vi "4_Speech_Rec_Deploy(mic).vi"() -> ()   [LabVIEW 2020]
doc: "This example demonstrates the usage of Deep Learning Toolkit for loading the model pretrained for objects recognition and running for inference."
uses:
  <vilib>/Ngene/Deep Learning Toolkit/Toolkit/NN_Network/Controls/NN_Device.ctl
  <vilib>/Ngene/Deep Learning Toolkit/Toolkit/NN_Network/Controls/NN_Save_Before_Destroy_Options.ctl
  <vilib>/sound2/lvsound2.llb/Sampling Mode.ctl
  <vilib>/sound2/lvsound2.llb/Sound Data Format.ctl
  <vilib>/Analysis/5stat.llb/RMS (DBL).vi
  <vilib>/sound2/lvsound2.llb/Sound Input Read (DBL).vi
  <vilib>/Ngene/Deep Learning Toolkit/Toolkit/NN_Network/API/NN_Set_Input/3D/NN_Set_Input(3D_SGL_idx).vi
  <vilib>/Ngene/Deep Learning Toolkit/Toolkit/Deep_Learning_Toolkit_by_Ngene.lvlib
  <vilib>/vision/NI_Vision_Development_Module.lvlib
  <vilib>/Analysis/NI_AALPro.lvlib
panel:
  out "Spectrogram":dbl[][](graph)
  out "Class Labels":string[](array[string])=["no", "stop", "down", "dog", "backward", "sheila", "zero", "visual", "wow", "left", "nine", "learn", "one", "go", "yes", "up", "follow", "four", "cat", "seven", "two", "_background_noise_", "off", "happy", "right", "bed", "marvin", "five", "six", "forward", "bird", "tree", "eight", "three", "house", "on"]
  out "Waveform":waveform(dbl)(graph)={"t0"=timestamp(3866543015.0437703 s since 1904-01-01), "dt"=6.25e-05, "Y"=array[16000 elements]}
  out "Class Probabilities":sgl[](array[slide])=[0.3439477, 0.21329805, 0.094255894, 0.046067823, 0.04473784, 0.04242303, 0.03942926, 0.036859456, 0.03191309, 0.028905181, 0.027009873, 0.013410927, 0.011738547, 0.0056317565, 0.005620018, 0.00169456, 0.00161148, 0.0014156047, 0.0013186012, 0.0013032081, 0.0012892308, 0.0008470631, 0.0008419843, 0.00080975075, 0.0006212335, 0.00061424717, 0.00059279194, 0.000582364, 0.00025428596, 0.00022874227, 0.0001889991, 0.00015415151, 0.00014091097, 0.00012097955, 6.820219e-05, 5.3142972e-05] scale=0.0..1.0
  in  "NN Device":T1=enum."GPU"
  out "Inference Time(sec)":dbl=0.012933300007716753 format="%#_3p"
  in  "Network Configuration File Path":path=path "D:/working/speech_rec/Speech_Rec_net_cfg_26_07_10__17_58_19.cfg"
  in  "Weight File Path":path=path "D:/working/speech_rec/Speech_Rec_weights_26_07_10__17_58_19.bin"
  in  "Stop":bool
  in  "threshold":dbl=0.01 format="%#_13g"
  # "Overview: This example demonstrates the use of Deep Learning Toolkit for loading a model pretrained for speech recognition and running it for inference.\nRequirements:\n1. Deep Learning Toolkit for LabVIEW.\n2. NI Vision Development Module.\n3. A PC with audio input (microphone).\nInstructions:\nThis example requires the trained model (network topology file .cfg and trained weights file .bin) generated in the previous step.\n1. Provide the trained model files at \"Network Configuration File Path\" and \"Weight File Path\".\n2. Run the VI.\n3. Pronounce one of the words from the dataset and observe the prediction results.\n4. Adjust the threshold value to reduce the false detection rate or increase sensitivity."
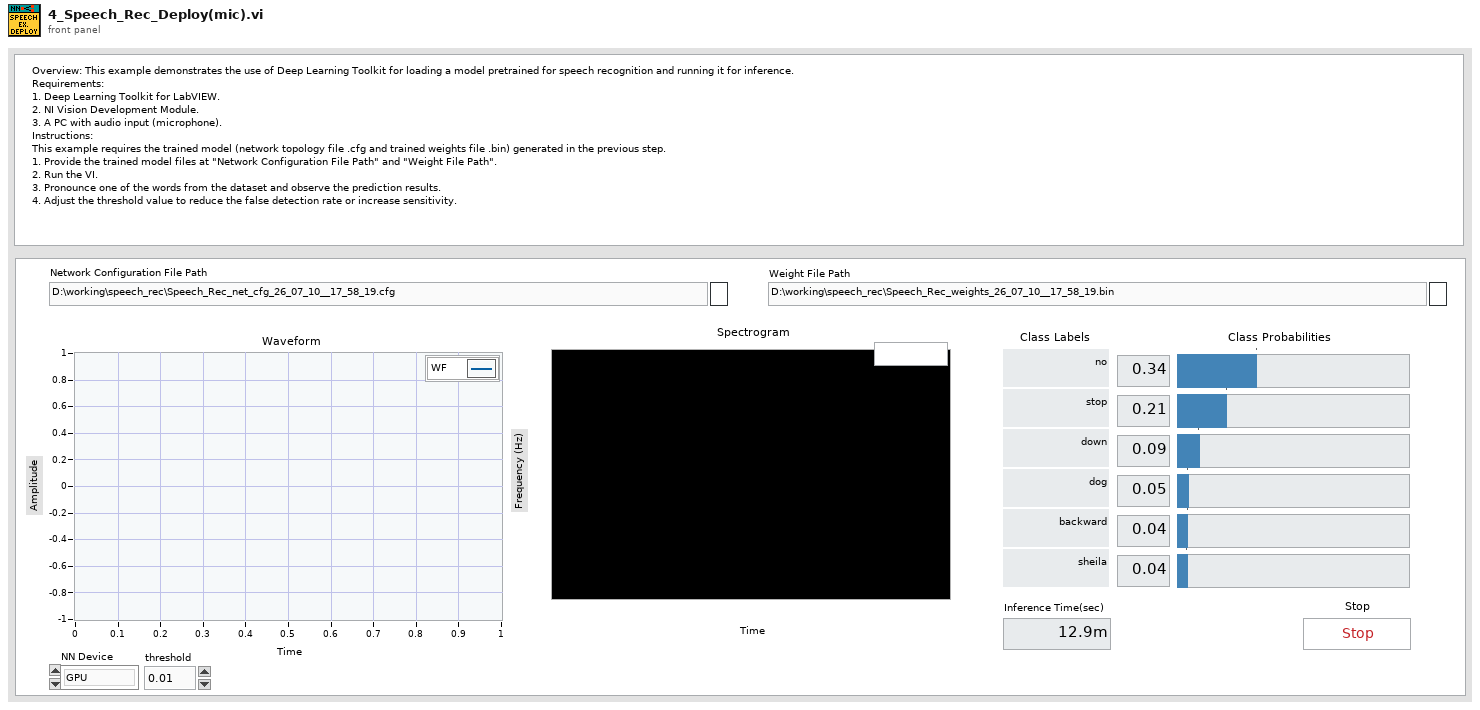
[diagram p1: front panel]
types:
  T1 = typedef "Deep_Learning_Toolkit_by_Ngene.lvlib/NN_Device.ctl" = enum16{"CPU", "GPU"}
  T2 = typedef "Sound Data Format.ctl" = cluster{"sample rate (S/s)":dbl, "number of channels":i32, "bits per sample":i32}
  T3 = typedef "Sampling Mode.ctl" = i32
  T4 = typedef "Image Type" = u32
  T5 = typedef "Deep_Learning_Toolkit_by_Ngene.lvlib/NN_Save_Before_Destroy_Options.ctl" = cluster{"CFG?":bool, "Weights?":bool, "Render?":bool}
  T6 = typedef "Sound Input Task ID.ctl" = u32
  T7 = typedef "Deep_Learning_Toolkit_by_Ngene.lvlib/NN_Config_Params.ctl" = cluster{"Name":string, "mBatch":i32, "NN_Train_Params":T8, "LR_Decay_Policy":T11, "Labels":string[], "Loss":T13, "Max_WS_Size(B)":i64, "DryRun?":bool}
  T8 = typedef "Deep_Learning_Toolkit_by_Ngene.lvlib/NN_Train_Params.ctl" = cluster{"Optimizer":T9, "Beta_1":sgl, "Beta_2":sgl, "Weight Decay(L1)":sgl, "Weight Decay(L2)":sgl, "Data_Sampling":T10}
  T9 = typedef "Deep_Learning_Toolkit_by_Ngene.lvlib/NN_Train_Optimizer.ctl" = enum16{"SGD", "Adam", "Adagrad", "Adadelta", "RMSProp", "Nesterov"}
  T10 = typedef "Deep_Learning_Toolkit_by_Ngene.lvlib/NN_Train_Data_Sampling.ctl" = enum16{"Random", "Sequential"}
  T11 = typedef "Deep_Learning_Toolkit_by_Ngene.lvlib/NN_LR_Policy_Cfg.ctl" = cluster{"Policy_Type":T12, "LR0":dbl, "k":sgl, "WarmUp_Policy":enum16{"Step", "Ramp"}, "WarmUp_Iter":i32, "WarmUp_Ratio":sgl}
  T12 = typedef "Deep_Learning_Toolkit_by_Ngene.lvlib/NN_LR_Policy_Type.ctl" = enum16{"Manual", "Step", "Exp", "1/t"}
  T13 = typedef "Deep_Learning_Toolkit_by_Ngene.lvlib/NN_Loss_Config_Params.ctl" = cluster{"Loss_Type":T14, "Loss_Conf_Params":variant}
  T14 = typedef "Deep_Learning_Toolkit_by_Ngene.lvlib/NN_Loss_Type.ctl" = enum16{"None", "MSE", "CrossEntropy", "YOLO_v2", "YOLO_v4"}
  T15 = typedef "Deep_Learning_Toolkit_by_Ngene.lvlib/NN_Layer_Config_Params.ctl" = cluster{"Layer_Type":T16, "Layer_Conf_Params":variant, "Input Layers":string[]}
  T16 = typedef "Deep_Learning_Toolkit_by_Ngene.lvlib/NN_Layer_Type.ctl" = enum16{"Input1D", "Input3D", "Conv1D", "Conv2D", "Conv2D_Adv", "MaxPool", "AvgPool", "UpSample", "DropOut3D", "ShortCut", "Concat", "SoftMax3D", "FC", "DropOut", "Softmax", "Flatten", "YOLO_v2", "YOLO_v4", "Activation", "BatchNormalization", "LayerNormalization", "Scale", "Unsupported"}
  T17 = typedef "Deep_Learning_Toolkit_by_Ngene.lvlib/NN.ctl" = cluster{"Name":string, "No of Layers":i32, "mBatch":i32, "Layers":T18[], "Dimty":T19, "Dims_In":T20, "Dims_Out":T20, "Working_Dir":path, "Train?":bool, "Train_Params":T8, "LR_Update_Policy":T11, "Session Data":T21, "Ground_truth":T22, "NNg_hdls":T23, "NN_Device":T1, "GPU Id":i32, "Labels":string[], "Loss_Type":T14, "Loss_Cfg_Prms":variant, "NNG_WS":T24, "DryRun?":bool}
  T18 = typedef "Deep_Learning_Toolkit_by_Ngene.lvlib/NN_Layer_ref.ctl" = refnum<file>
  T19 = typedef "Deep_Learning_Toolkit_by_Ngene.lvlib/NN_In_Out_Dim-ty.ctl" = enum8{"In1D_Out1D", "In3D_Out1D", "In3D_Out3D", "In3D_OutBBox"}
  T20 = typedef "Deep_Learning_Toolkit_by_Ngene.lvlib/NN_Dims(C,H,W).ctl" = cluster{"C":i32, "H":i32, "W":i32}
  T21 = typedef "Deep_Learning_Toolkit_by_Ngene.lvlib/NN_Train_Session_Data.ctl" = cluster{"Epochs":sgl, "Tot_Iter":i32, "LR":sgl, "LR_iter":i32}
  T22 = typedef "Deep_Learning_Toolkit_by_Ngene.lvlib/NN_Ground_truth.ctl" = cluster{"Y":variant}
  T23 = typedef "Deep_Learning_Toolkit_by_Ngene.lvlib/nng_cuda_handles.ctl" = cluster{"cudnn":u64, "cublas":u64, "stream":u64, "curand":u64}
  T24 = typedef "Deep_Learning_Toolkit_by_Ngene.lvlib/NNG_WS.ctl" = cluster{"NNG_WS_Mem":T25, "Max_WS_Size":i64}
  T25 = typedef "Deep_Learning_Toolkit_by_Ngene.lvlib/NNg_WS_Mem_DVR.ctl" = refnum<data-value>
  T26 = typedef "IMAQ Image.ctl" = refnum<image>
  T27 = cluster{"spectral map":dbl[][], "X scale":cluster{"offset":dbl, "multiplier":dbl}, "Y scale":cluster{"offset":dbl, "multiplier":dbl}, "attribute":variant}
  T28 = typedef "Deep_Learning_Toolkit_by_Ngene.lvlib/NN_Layer.ctl" = cluster{"Name":string, "Layer_Data":T29, "Layer_Type":T16, "Dims_In":T20, "Layers_In":T18[], "Dims_Out":T20, "Layers_Out":T18[], "Metrics":T30, "GPU_Data":T31, "mBatch":i32, "NN_Device":T1, "NNg_hdls":T23, "Train?":bool, "Dimty":T32, "RecptField":T33, "Idx":i32}
  T29 = typedef "Deep_Learning_Toolkit_by_Ngene.lvlib/NN_Layer_Data_Refnum.ctl" = refnum<file>
  T30 = typedef "Deep_Learning_Toolkit_by_Ngene.lvlib/NN_Layer_Metrics.ctl" = cluster{"Data":dbl, "Params":dbl, "Ops":dbl}
  T31 = typedef "Deep_Learning_Toolkit_by_Ngene.lvlib/NNg_Layer_Data_Refnum.ctl" = refnum<file>
  T32 = typedef "Deep_Learning_Toolkit_by_Ngene.lvlib/NN_Layer_Dimty.ctl" = enum16{"1D", "3D"}
  T33 = typedef "Deep_Learning_Toolkit_by_Ngene.lvlib/NN_Layer_RF_State.ctl" = cluster{"Dims":T34, "J":T34}
  T34 = typedef "Deep_Learning_Toolkit_by_Ngene.lvlib/NN_Dims(V,H).ctl" = cluster{"V":i32, "H":i32}
  T35 = cluster{"Numeric Control":sgl, "Labels":string}[]
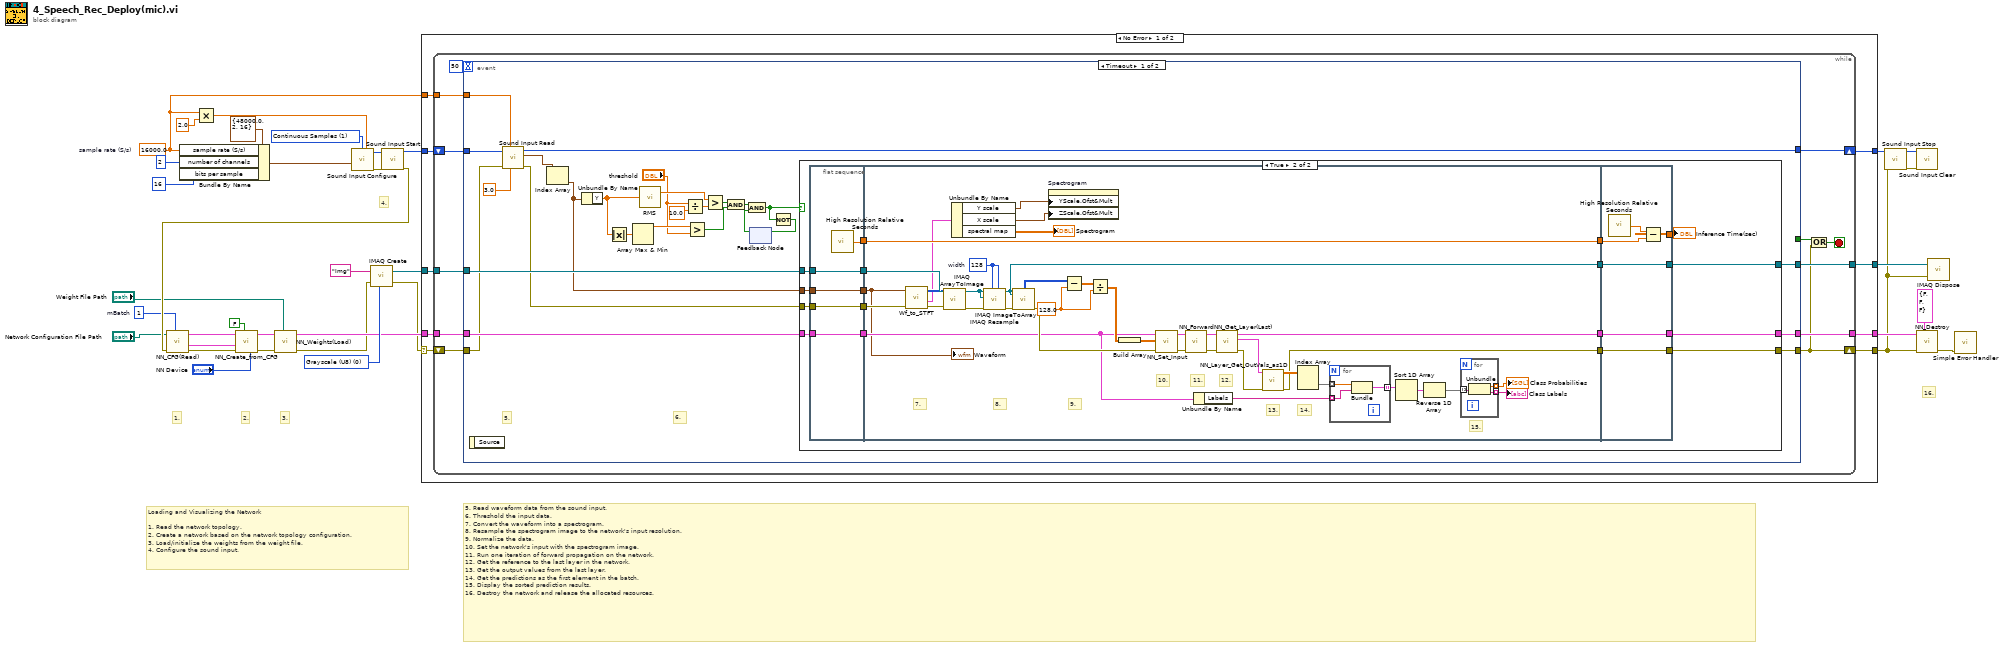
[diagram p0: block diagram]
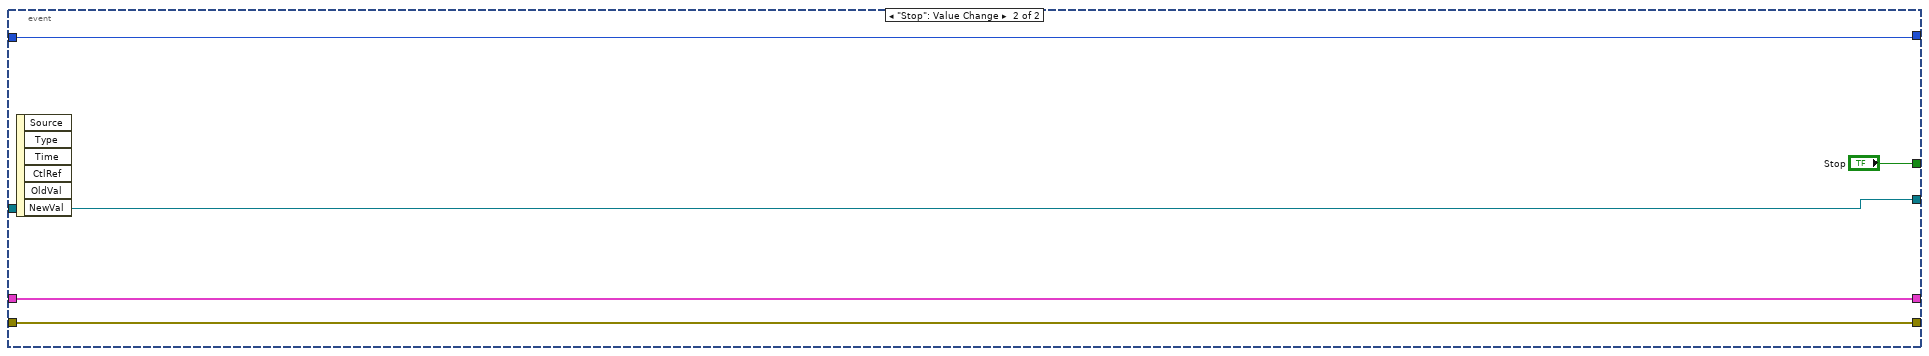
[diagram p3: hidden frame]
diagram:
  w4 = 1  # mBatch
  w9 = 16000.0  # sample rate (S/s)
  w18 = T3 1 items=["Finite Samples", "Continuous Samples"] ("sample mode")
  w32 = T4 0 items=["Grayscale (U8)", "Grayscale (I16)", "Grayscale (SGL)", "Complex (CSG)", "RGB (U32)", "HSL (U32)", "RGB (U64)", "Grayscale (U16)"] ("Image Type")
  # "16."
  # "5. Read waveform data from the sound input.\n6. Threshold the input data.\n7. Convert the waveform into a spectrogram.\n8. Resample the spectrogram image to the network's input resolution.\n9. Normalize the data.\n10. Set the network's input with the spectrogram image.\n11. Run one iteration of forward propagation on the network.\n12. Get the reference to the last layer in the network.\n13. Get the output values from the last layer.\n14. Get the predictions as the first element in the batch.\n15. Display the sorted prediction results.\n16. Destroy the network and release the allocated resources."
  # "4."
  # "3."
  # "2."
  # "1."
  # "Loading and Visualizing the Network\n\n1. Read the network topology.\n2. Create a network based on the network topology configuration.\n3. Load/initialize the weights from the weight file.\n4. Configure the sound input."
  n1 = Bundle By Name(cluster=T2 {"sample rate (S/s)"=48000.0, "number of channels"=2, "bits per sample"=16} ("sound format"), "sample rate (S/s)"=w9, "number of channels"=2, "bits per sample"=16) -> (w20:T2)
  n2 = Multiply(x=w9, y=2.0 ("x")) -> (x*y=w10:dbl)
  n3 = call <vilib>:"Sound Input Configure.vi"("number of samples/ch"=w10, "sample mode"=w18, "sound format"=w20) -> ("error out"=w17:errorcluster, "task ID"=w16:T6)  [unwired: 7 in]
  n4 = call <vilib>:"Sound Input Start.vi"("error in (no error)"=w17, "task ID"=w16) -> ("error out"=w6:errorcluster, "task ID out"=w15:T6)  [unwired: 8 in]
  n5 = call <vilib>:"NN_CFG(Read).vi"("mBatch"=w4, "error in (no error)"=w6, "CFG file path"="Network Configuration File Path") -> ("error out"=w30:errorcluster, "Net_Cfg"=w29:T7, "Layer_Cfg"=w8:T15[])  [unwired: 6 in]
  n6 = call <vilib>:"NN_Create_from_CFG.vi"("NN_Device"="NN Device", "Train? (false)"=FALSE, "error in (no error)"=w30, "Net_Cfg"=w29, "Layer_Cfg"=w8) -> ("error out"=w28:errorcluster, "NN out"=w7:T17)  [unwired: 5 in]
  n7 = call <vilib>:"NN_Weights(Load).vi"("Weight File Path"="Weight File Path", "error in (no error)"=w28, "NN in"=w7) -> ("error out"=w24:errorcluster, "NN out"=w27:T17)  [unwired: 7 in]
  n8 = call "IMAQ Create"("Image Name"="Img", "Image Type"=w32, "error in (no error)"=w24) -> ("New Image"=w31:T26, "error out"=w23:errorcluster)  [unwired: 2 in]
  n9 = case shown="No Error" w23 {
    selector: w23 -> [w44 w165]
    tunnel: w27 -> [w42 w167]
    tunnel: [w45 w167] -> w34
    tunnel: [w37 w165] -> w5
    tunnel: w31 -> [w43 w166]
    tunnel: [w41 w166] -> w26
    tunnel: w15 -> [w40 w164]
    tunnel: [w39 w164] -> w12
    tunnel: w9 -> [w38 _]
    frame No Error {
      n10 = while {
        tunnel: [w54] -> w45
        tunnel: w43 -> [w56]
        tunnel: w42 -> [w55]
        tunnel: [w53] -> w41
        shift-right: [w51] -> w39
        shift-left: w40 -> [w52]
        tunnel: w38 -> [w50]
        shift-right: [w47] -> w37
        shift-left: w44 -> [w57]
        stop <- w49 stop-if-true
        n11 = event shown="[0] Timeout" {
          selector: _ -> [_ _]
          dyn-events: _ -> [_ _]
          timeout: 50 -> [_ _]
          tunnel: w57 -> [w71 w161]
          tunnel: w56 -> [w83 w160]
          tunnel: w55 -> [w82 w162]
          tunnel: [w81 w162] -> w54
          tunnel: [w80 w160] -> w53
          tunnel: w52 -> [w78 w163]
          tunnel: [w77 w163] -> w51
          tunnel: [w75 w161] -> w47
          tunnel: w50 -> [w72 _]
          tunnel: [_ "Stop"] -> w48
          event Timeout {
            # "6."
            # "5."
            n12 = event-data() -> ()  [unwired: 1 in, 1 out]
            n13 = call-poly <vilib>:"Sound Input Read.vi"("timeout (sec)"=3.0, "number of samples/ch"=w72, "error in (no error)"=w71, "task ID"=w78) -> ("error out"=w70:errorcluster, "data"=w79:waveform(dbl)[], "task ID out"=w77:T6)  [unwired: 5 in]
            n14 = Index Array(array=w79) -> (element=w58:waveform(dbl))  [unwired: 1 in]
            n15 = Unbundle By Name(w58) -> ("Y"=w66:dbl[])
            n16 = Absolute Value(x=w66) -> (abs(x)=w62:dbl[])
            n17 = Array Max & Min(array=w62) -> (max value=w68:dbl)  [unwired: 3 out]
            n18 = call-poly <vilib>:"RMS.vi"("X"=w66) -> ("rms value"=w76:dbl)  [unwired: 1 out]
            n19 = Divide(x="threshold", y=10.0) -> (x/y=w65:dbl)
            n20 = Greater?(x=w68, y="threshold") -> (0:w67:bool)
            n21 = Greater?(x=w76, y=w65) -> (0:w74:bool)
            n22 = And(x=w74, y=w67) -> (x .and. y?=w69:bool)
            n23 = feedback #1() -> (w59:bool)  [unwired: 1 in]
            n24 = And(x=w69, y=w59) -> (x .and. y?=w61:bool)
            n25 = Not(x=w61) -> (.not. x?=w60:bool)
            n26 = feedback-in #1(w60) -> ()
            n27 = case shown="True" w61 {
              tunnel: w70 -> [w84 w97]
              tunnel: w83 -> [w86 w103]
              tunnel: w82 -> [w85 w102]
              tunnel: [w85 w101] -> w81
              tunnel: [w86 w100] -> w80
              tunnel: [w84 w99] -> w75
              tunnel: w58 -> [_ w98]
              frame False {
              }
              frame True {
                n28 = flat-sequence {
                  tunnel: w97 -> [w105]
                  tunnel: w98 -> [w106]
                  tunnel: w102 -> [w107]
                  tunnel: w103 -> [w108]
                  tunnel: [w108] -> w96
                  tunnel: [w107] -> w95
                  tunnel: [w106] -> w94
                  tunnel: [w105] -> w93
                  tunnel: [w104] -> w89
                  tunnel: w96 -> [w146]
                  tunnel: w95 -> [w119]
                  tunnel: w94 -> [w112]
                  tunnel: w93 -> [w133]
                  tunnel: [w145] -> w92
                  tunnel: [w144] -> w91
                  tunnel: [w136] -> w90
                  tunnel: w89 -> [w123]
                  tunnel: [w123] -> w88
                  tunnel: [w156] -> w99
                  tunnel: [w157] -> w100
                  tunnel: [w158] -> w101
                  tunnel: w92 -> [w158]
                  tunnel: w91 -> [w157]
                  tunnel: w90 -> [w156]
                  tunnel: w88 -> [w154]
                  tunnel: [w153] -> w87
                  frame #0 {
                    n29 = call <vilib>:"High Resolution Relative Seconds.vi"() -> ("relative seconds"=w104:dbl)
                  }
                  frame #1 {
                    w122 = sgl 128.0 ("dimension size")
                    w120 = 128  # width
                    # "15."
                    # "14."
                    # "13."
                    # "12."
                    # "11."
                    # "10."
                    # "9."
                    # "8."
                    # "7."
                    n30 = call "Wf_to_STFT.vi"("error in (no error)"=w133, "WF"=w112) -> ("error out"=w134:errorcluster, "STFT"=w114:T27, "Image_data"=w135:u8[][])  [unwired: 7 in]
                    n31 = call "IMAQ ArrayToImage"("error in (no error)"=w134, "Image Pixels (U8)"=w135, "Image"=w146) -> ("error out"=w138:errorcluster, "Image Out"=w139:T26)  [unwired: 7 in]
                    n32 = Unbundle By Name(w114) -> ("Y scale"=w116:cluster{"offset":dbl, "multiplier":dbl}, "X scale"=w115:cluster{"offset":dbl, "multiplier":dbl}, "spectral map"=→"Spectrogram":dbl[][])
                    n33 = call "IMAQ Resample"("X Resolution"=w120, "Y Resolution"=w120, "error in (no error)"=w138, "Image Dst"=w139, "Image Src"=w139) -> ("error out"=w137:errorcluster, "Image Dst Out"=w144:T26)  [unwired: 5 in]
                    n34 = call "IMAQ ImageToArray"("error in (no error)"=w137, "Image"=w144) -> ("error out"=w132:errorcluster, "Image Pixels (U8)"=w121:u8[][])  [unwired: 2 in, 3 out]
                    n35 = property on="Spectrogram" class="IntGraph (strict)"("YScale.Ofst&Mult"=w116, "ZScale.Ofst&Mult"=w115) -> ()  [unwired: 2 in, 2 out]
                    n36 = Subtract(x=w121, y=w122) -> (x-y=w125:sgl[][])
                    n37 = Divide(x=w125, y=w122) -> (x/y=w124:sgl[][])
                    n38 = Build Array(w124) -> (w117:sgl[][][])
                    n39 = call-poly <vilib>:"NN_Set_Input.vi"("error in (no error)"=w132, "Data_In(3D_SGL)"=w117, "NN in"=w119) -> ("error out"=w129:errorcluster, "NN out"=w128:T17)  [unwired: 7 in]
                    n40 = call <vilib>:"NN_Forward.vi"("error in (no error)"=w129, "NN in"=w128) -> ("error out"=w127:errorcluster, "NN out"=w126:T17)  [unwired: 6 in, 2 out]
                    n41 = Unbundle By Name(w119) -> ("Labels"=w118:string[])
                    n42 = call <vilib>:"NN_Get_Layer(Last).vi"("error in (no error)"=w127, "NN in"=w126) -> ("error out"=w131:errorcluster, "Last_Layer"=w130:T28, "NN out"=w145:T17)  [unwired: 6 in, 1 out]
                    n43 = call <vilib>:"NN_Layer_Get_OutVals_as1D.vi"("error in (no error)"=w131, "Layer"=w130) -> ("error out"=w136:errorcluster, "Out(as1D)"=w143:sgl[][])  [unwired: 8 in]
                    n44 = Index Array(array=w143) -> (element=w140:sgl[])  [unwired: 2 in]
                    n45 = for {
                      tunnel: w140 -> [w152] mode=indexing
                      tunnel: w118 -> [w151] mode=indexing
                      tunnel: [w150] -> w142 mode=indexing
                      n46 = Bundle("Numeric Control"=w152, "Labels"=w151) -> (w150:cluster{"Numeric Control":sgl, "Labels":string})  [unwired: 1 in]
                    }
                    n47 = Sort 1D Array(array=w142) -> (sorted array=w141:T35)
                    n48 = Reverse 1D Array(array=w141) -> (reversed array=w111:T35)
                    n49 = for {
                      tunnel: w111 -> [w149] mode=indexing
                      tunnel: [w148] -> w109 mode=indexing
                      tunnel: [w147] -> w110 mode=indexing
                      n50 = Unbundle(w149) -> ("Numeric Control"=w148:sgl, "Labels"=w147:string)
                    }
                    "Class Probabilities" <- w109
                    "Class Labels" <- w110
                    "Waveform" <- w112
                  }
                  frame #2 {
                    n51 = call <vilib>:"High Resolution Relative Seconds.vi"() -> ("relative seconds"=w155:dbl)
                    n52 = Subtract(x=w155, y=w154) -> (x-y=w153:dbl)
                  }
                }
                "Inference Time(sec)" <- w87
              }
            }
          }
          event "Stop": Value Change {
            n53 = event-data() -> ()  [unwired: 1 in, 6 out]
          }
        }
        n54 = Or(x=w48, y=w47) -> (x .or. y?=w49:bool)
      }
    }
    frame Error {
    }
  }
  n55 = call <vilib>:"Sound Input Stop.vi"("error in (no error)"=w5, "task ID"=w12) -> ("error out"=w14:errorcluster, "task ID out"=w13:T6)  [unwired: 8 in]
  n56 = call <vilib>:"Sound Input Clear.vi"("error in (no error)"=w14, "task ID"=w13) -> ()  [unwired: 9 in, 1 out]
  n57 = call <vilib>:"NN_Destroy.vi"("Save (T, T, T)"=T5 {"CFG?"=FALSE, "Weights?"=FALSE, "Render?"=FALSE} ("Save_Config"), "error in (no error)"=w5, "NN in"=w34) -> ("error out"=w36:errorcluster)  [unwired: 7 in, 1 out]
  n58 = call "IMAQ Dispose"("Image"=w26, "error in (no error)"=w5) -> ()  [unwired: 4 in, 1 out]
  n59 = call <vilib>:"Simple Error Handler.vi"("error in (no error)"=w36) -> ()  [unwired: 4 in, 5 out]
